vi "get HovaCAL Sollwerte je MFC.vi"(10 "MFC in":u32, 11 "Sollwert je MFC Cluster":T1) -> (3 "Sollwert MFC":sgl[](array[numeric]))   [LabVIEW 2020, in "Linearisierung v2.lvlib"]
uses:
  Linearisierung v2.lvlib
  HovaCAL Sollwerte je MFC Cluster.ctl
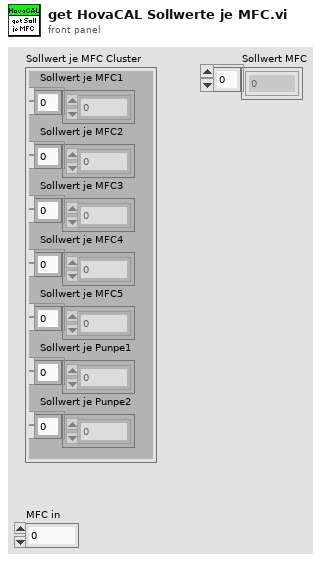
[diagram p1: front panel]
types:
  T1 = typedef "Linearisierung v2.lvlib/HovaCAL Sollwerte je MFC Cluster.ctl" = cluster{"Sollwert je MFC1":sgl[], "Sollwert je MFC2":sgl[], "Sollwert je MFC3":sgl[], "Sollwert je MFC4":sgl[], "Sollwert je MFC5":sgl[], "Sollwert je Punpe1":sgl[], "Sollwert je Punpe2":sgl[]}
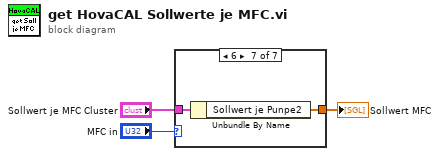
[diagram p0: block diagram]
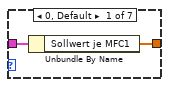
[diagram p2: hidden frame]
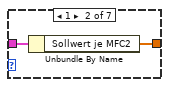
[diagram p3: hidden frame]
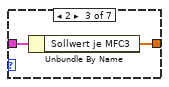
[diagram p4: hidden frame]
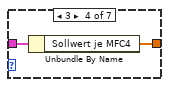
[diagram p5: hidden frame]
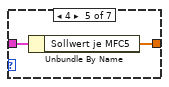
[diagram p6: hidden frame]
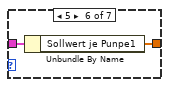
[diagram p7: hidden frame]
diagram:
  n1 = case shown="6" "MFC in" {
    tunnel: "Sollwert je MFC Cluster" -> [w5 w7 w9 w11 w13 w15 w17]
    tunnel: [w4 w6 w8 w10 w12 w14 w16] -> w1
    frame 0, Default {
      n2 = Unbundle By Name(w5) -> ("Sollwert je MFC1"=w4:sgl[])
    }
    frame 1 {
      n3 = Unbundle By Name(w7) -> ("Sollwert je MFC2"=w6:sgl[])
    }
    frame 2 {
      n4 = Unbundle By Name(w9) -> ("Sollwert je MFC3"=w8:sgl[])
    }
    frame 3 {
      n5 = Unbundle By Name(w11) -> ("Sollwert je MFC4"=w10:sgl[])
    }
    frame 4 {
      n6 = Unbundle By Name(w13) -> ("Sollwert je MFC5"=w12:sgl[])
    }
    frame 5 {
      n7 = Unbundle By Name(w15) -> ("Sollwert je Punpe1"=w14:sgl[])
    }
    frame 6 {
      n8 = Unbundle By Name(w17) -> ("Sollwert je Punpe2"=w16:sgl[])
    }
  }
  "Sollwert MFC" <- w1
